vi "Read JSON reader.lvclass.vi"(8 "error in (no error)":errorcluster, 11 "File interpreter in":refnum<class "File interpreter.lvclass">) -> (0 "error out":errorcluster, 2 "JSON reader.lvclass":refnum<class "JSON reader.lvclass">, 3 "File interpreter out":refnum<class "File interpreter.lvclass">)   [LabVIEW 2018, in "File interpreter.lvclass"]
uses:
  File interpreter.lvclass
  JSON reader/JSON reader.lvclass
  File interpreter.lvclass/File interpreter.ctl
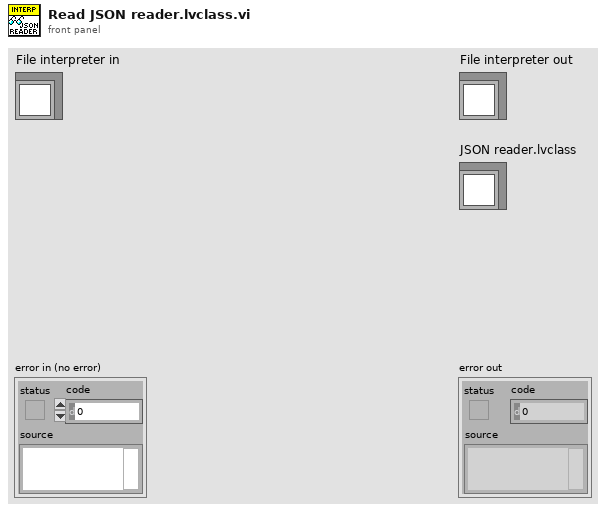
[diagram p1: front panel]
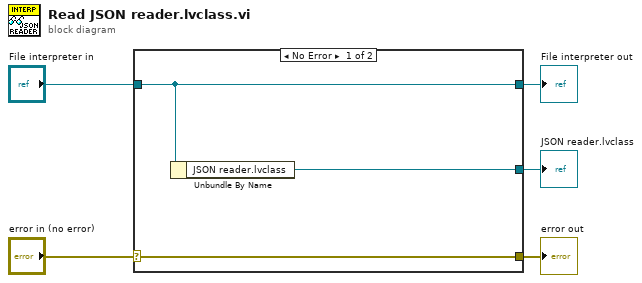
[diagram p0: block diagram]
diagram:
  n1 = case shown="No Error" "error in (no error)" {
    selector: "error in (no error)" -> [w8 w9]
    tunnel: [w8 w9] -> w4
    tunnel: [w7 w10] -> w2
    tunnel: "File interpreter in" -> [w7 w10]
    tunnel: [w6 _] -> w1
    frame No Error {
      n2 = Unbundle By Name(w7) -> ("JSON reader.lvclass"=w6:refnum<class "JSON reader.lvclass">)
    }
    frame Error {
    }
  }
  "error out" <- w4
  "File interpreter out" <- w2
  "JSON reader.lvclass" <- w1
